vi "temperature.vi"() -> (0 "Actual Temp":dbl)   [LabVIEW 2013]
uses:
  <vilib>/Analysis/NI_AALBase.lvlib
panel:
  out "Temperature":dbl(graph)
  out "Start Temp":dbl
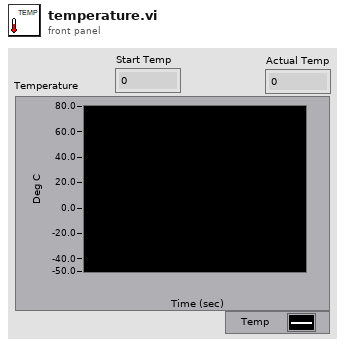
[diagram p1: front panel]
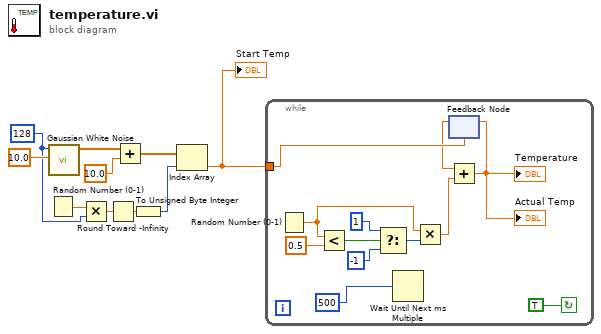
[diagram p0: block diagram]
diagram:
  w6 = 128
  n1 = Random Number (0-1)() -> (number: 0 to 1=w7:dbl)
  n2 = call <vilib>:"Gaussian White Noise.vi"("standard deviation"=10.0, "samples"=w6) -> ("Gaussian noise pattern"=w10:dbl[])  [unwired: 8 in, 1 out]
  n3 = Multiply(x=w7, y=w6) -> (x*y=w5:dbl)
  n4 = Round Toward -Infinity(1:w5) -> (0:w4:dbl)
  n5 = Add(x=w10, y=10.0) -> (x+y=w2:dbl[])
  n6 = To Unsigned Byte Integer(number=w4) -> (unsigned 8bit integer=w3:u8)
  n7 = Index Array(array=w2, index=w3) -> (element=w1:dbl)
  "Start Temp" <- w1
  n8 = while {
    tunnel: w1 -> [w13]
    stop <- TRUE continue-if-true
    n9 = Random Number (0-1)() -> (number: 0 to 1=w16:dbl)
    n10 = Less?(x=w16, y=0.5) -> (x < y?=w21:bool)
    n11 = Select(t=1, s=w21, f=-1) -> (s? t:f=w17:i32)
    n12 = Wait Until Next ms Multiple(millisecond multiple=500) -> ()  [unwired: 1 out]
    n13 = Multiply(x=w16, y=w17) -> (x*y=w15:dbl)
    n14 = feedback #1(w13) -> (w12:dbl)
    n15 = Add(x=w12, y=w15) -> (x+y=w11:dbl)
    "Temperature" <- w11
    "Actual Temp" <- w11
    n16 = feedback-in #1(w11) -> ()
  }
